vi "pharosTriggersDoubleTrainGenerateBoolLines.vi"(1 "off at the end":bool=TRUE, 2 "time btwn trains (s)":dbl, 3 "n trains":i32) -> (0 "triggers":u8[](array[numeric]))   [LabVIEW 2017]
uses:
  globalUtilities.vi
  globalDevices.vi
panel:
  out "x-y":dbl
  out "size(s)":i32
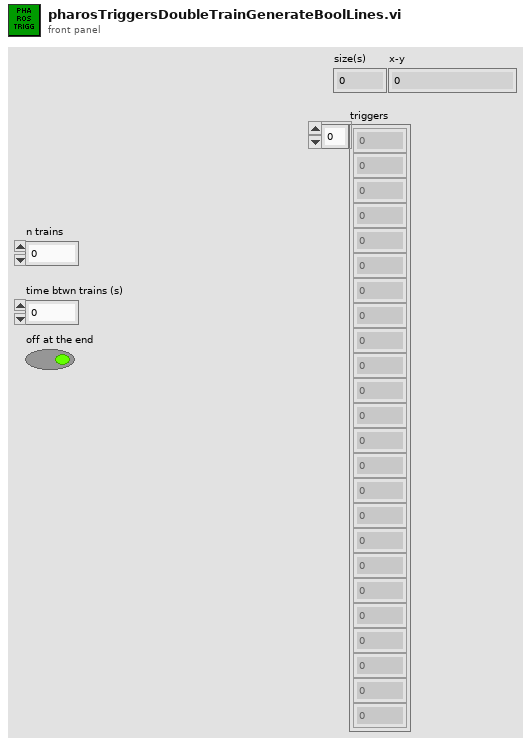
[diagram p1: front panel]
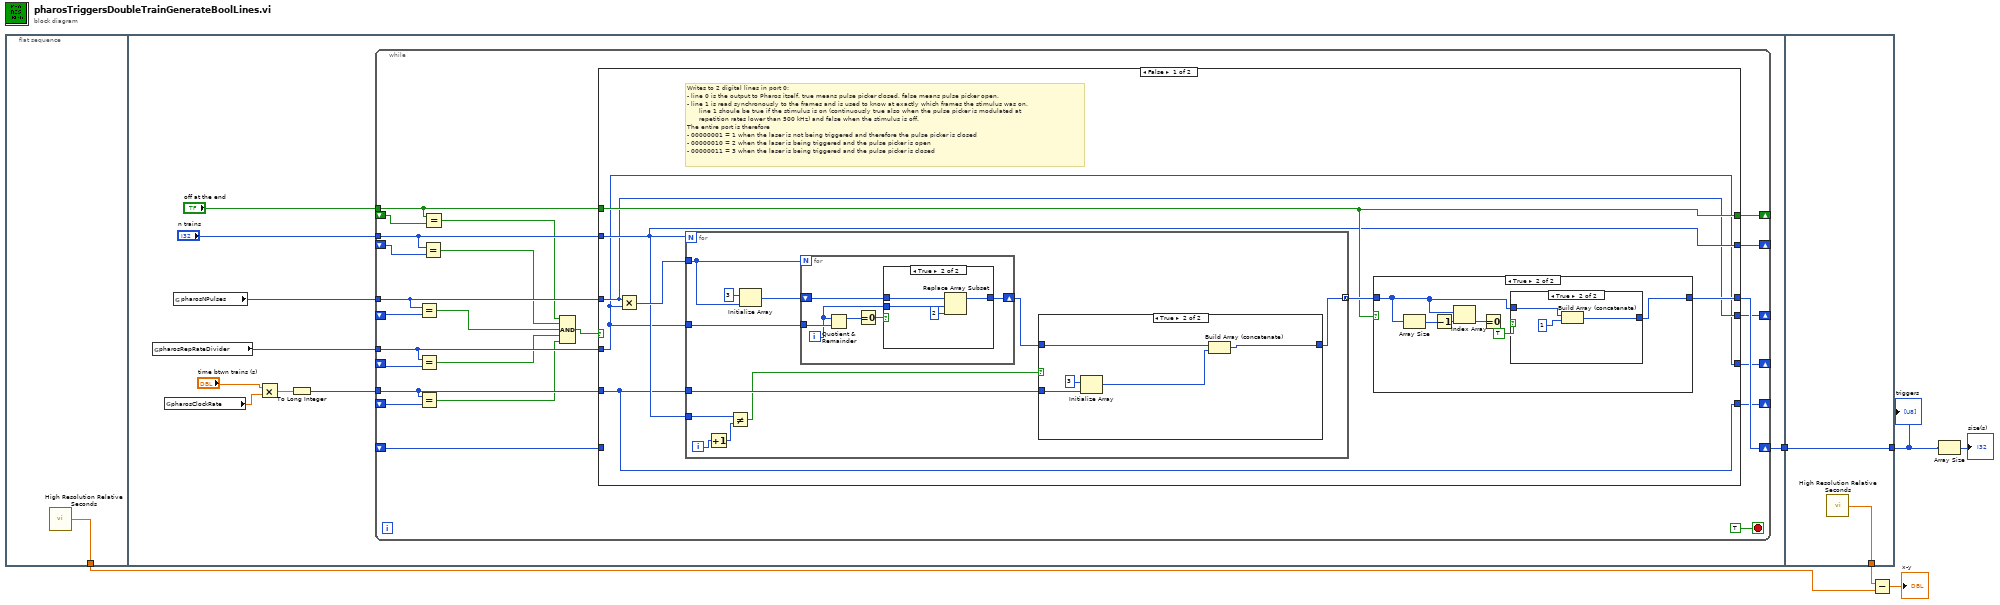
[diagram p0: block diagram]
diagram:
  n1 = flat-sequence {
    tunnel: [w7] -> w2
    tunnel: [w13] -> w4
    tunnel: [w95] -> w6
    tunnel: w4 -> [w95]
    tunnel: [w94] -> w3
    frame #0 {
      n2 = call <vilib>:"High Resolution Relative Seconds.vi"() -> ("relative seconds"=w7:dbl)
    }
    frame #1 {
      n3 = global read "globalUtilities.vi" "pharosRepRateDivider"() -> (w16:i32)
      n4 = global read "globalDevices.vi" "pharosClockRate"() -> (w10:dbl)
      n5 = global read "globalUtilities.vi" "pharosNPulses"() -> (w15:i32)
      n6 = Multiply(x="time btwn trains (s)", y=w10) -> (x*y=w9:dbl)
      n7 = To Long Integer(number=w9) -> (32bit integer=w8:i32)
      n8 = while {
        tunnel: w16 -> [w28]
        tunnel: w15 -> [w30]
        tunnel: "off at the end" -> [w34]
        tunnel: "n trains" -> [w32]
        tunnel: w8 -> [w26]
        shift-right: [w39] -> _
        shift-left: _ -> [w33]
        shift-right: [w38] -> _
        shift-left: _ -> [w31]
        shift-right: [w37] -> _
        shift-left: _ -> [w29]
        shift-right: [w36] -> _
        shift-left: _ -> [w27]
        shift-right: [w35] -> _
        shift-left: _ -> [w25]
        shift-right: [w40] -> w13
        shift-left: _ -> [w18]
        stop <- TRUE stop-if-true
        n9 = Equal?(x=w28, y=w27) -> (x = y?=w21:bool)
        n10 = Equal?(x=w30, y=w29) -> (x = y?=w22:bool)
        n11 = Equal?(x=w26, y=w25) -> (x = y?=w20:bool)
        n12 = Equal?(x=w32, y=w31) -> (x = y?=w23:bool)
        n13 = Equal?(x=w34, y=w33) -> (x = y?=w24:bool)
        n14 = Compound Arithmetic op=AND(w24, w23, w22, w21, w20) -> (w19:bool)
        n15 = case shown="False" w19 {
          tunnel: w28 -> [w42 w90]
          tunnel: w30 -> [w43 w91]
          tunnel: w34 -> [w45 w93]
          tunnel: [w46 w88] -> w40
          tunnel: w32 -> [w44 w92]
          tunnel: w26 -> [w41 w89]
          tunnel: [w45 w93] -> w39
          tunnel: [w44 w92] -> w38
          tunnel: [w43 w91] -> w37
          tunnel: [w42 w90] -> w36
          tunnel: [w41 w89] -> w35
          tunnel: w18 -> [_ w88]
          frame False {
            # "Writes to 2 digital lines in port 0:\n- line 0 is the output to Pharos itself. true means pulse picker closed, false means pulse picker open.\n- line 1 is read synchronously to the frames and is used to know at exactly which frames the stimulus was on.\n      line 1 shoule be true if the stimulus is on (continuously true also when the pulse picker is modulated at\n      repetition rates lower than 500 kHz) and false when the stimulus is off.\nThe entire port is therefore\n- 00000001 = 1 when the laser is not being triggered and therefore the pulse picker is closed\n- 00000010 = 2 when the laser is being triggered and the pulse picker is open\n- 00000011 = 3 when the laser is being triggered and the pulse picker is closed"
            n16 = Multiply(x=w43, y=w42) -> (x*y=w48:i32)
            n17 = for {
              N: w44 -> [_]
              tunnel: w42 -> [w57]
              tunnel: w48 -> [w56]
              tunnel: [w49] -> w47 mode=concatenating
              tunnel: w44 -> [w53]
              tunnel: w41 -> [w52]
              i -> [w55]
              n18 = Increment(x=w55) -> (x+1=w54:i32)
              n19 = Not Equal?(x=w53, y=w54) -> (x != y?=w51:bool)
              n20 = Initialize Array(u8 3 ("element"), w56) -> (w58:u8[])
              n21 = for {
                N: w56 -> [_]
                tunnel: w57 -> [w70]
                shift-right: [w66] -> w50
                shift-left: w58 -> [w71]
                i -> [w67]
                n22 = Quotient & Remainder(x=w67, y=w70) -> (x-y*floor(x/y)=w69:i32)  [unwired: 1 out]
                n23 = Equal To 0?(x=w69) -> (x = 0?=w68:bool)
                n24 = case shown="True" w68 {
                  tunnel: w71 -> [w72 w76]
                  tunnel: w67 -> [_ w75]
                  tunnel: [w72 w73] -> w66
                  frame False {
                  }
                  frame True {
                    n25 = Replace Array Subset(array=w76, new element=u8 2 ("new element/subarray"), index=w75) -> (w73:u8[])
                  }
                }
              }
              n26 = case shown="True" w51 {
                tunnel: w52 -> [_ w64]
                tunnel: w50 -> [w60 w63]
                tunnel: [w60 w61] -> w49
                frame False {
                }
                frame True {
                  n27 = Initialize Array(u8 3 ("element"), w64) -> (w62:u8[])
                  n28 = Build Array (concatenate)(w63, w62) -> (w61:u8[])
                }
              }
            }
            n29 = case shown="True" w45 {
              tunnel: w47 -> [w77 w81]
              tunnel: [w77 w80] -> w46
              frame False {
              }
              frame True {
                n30 = Array Size(array=w81) -> (size(s)=w82:i32)
                n31 = Decrement(x=w82) -> (x-1=w79:i32)
                n32 = Index Array(array=w81, index=w79) -> (element=w83:u8)
                n33 = Equal To 0?(x=w83) -> ()  [unwired: 1 out]
                n34 = case shown="True" TRUE {
                  tunnel: w81 -> [w84 w87]
                  tunnel: [w84 w85] -> w80
                  frame False {
                  }
                  frame True {
                    n35 = Build Array (concatenate)(w87, u8 1) -> (w85:u8[])
                  }
                }
              }
            }
          }
          frame True {
          }
        }
      }
    }
    frame #2 {
      n36 = call <vilib>:"High Resolution Relative Seconds.vi"() -> ("relative seconds"=w94:dbl)
    }
  }
  n37 = Subtract(x=w3, y=w2) -> (x-y=→"x-y":dbl)
  n38 = Array Size(array=w6) -> (size(s)=→"size(s)":i32)
  "triggers" <- w6
